vi "JSON Key Search.vi"(9 "offset (0)":i32, 10 "Key":string, 11 "JSON":string) -> (1 "offset of match":i32, 2 "JSON Type":T1, 3 "Value":string)   [LabVIEW 2013, in "LV JSON.lvlib"]
doc: "Search JSON string for Key name and return corresponding value and the JSON type of the value."
uses:
  LV JSON.lvlib
  controls/JSON type.ctl
  <vilib>/Utility/error.llb/Trim Whitespace.vi
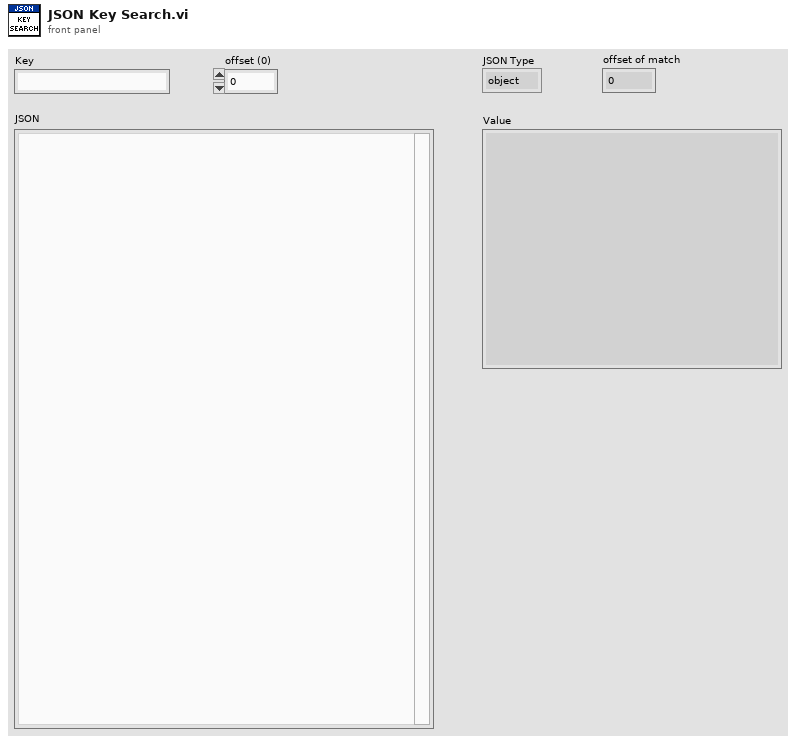
[diagram p1: front panel]
types:
  T1 = typedef "LV JSON.lvlib/JSON type.ctl" = enum16{"object", "array", "number", "string", "boolean", "null"}
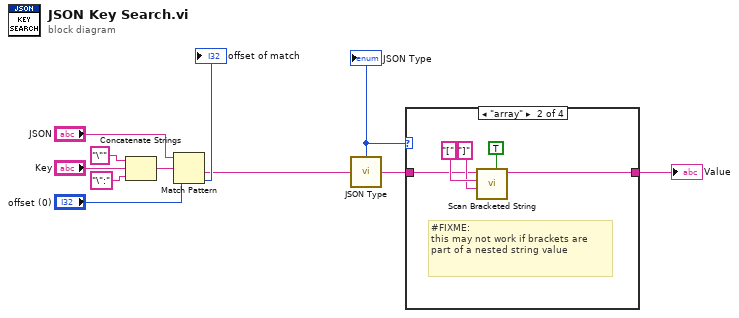
[diagram p0: block diagram]
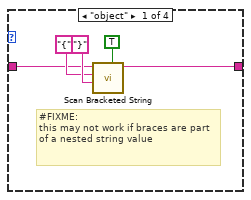
[diagram p2: hidden frame]
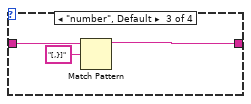
[diagram p3: hidden frame]
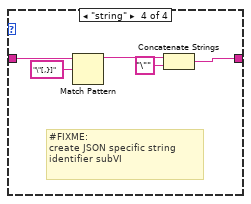
[diagram p4: hidden frame]
diagram:
  n1 = Concatenate Strings("\"" ("string"), "Key", "\":" ("string")) -> (w8:string)
  n2 = Match Pattern(string="JSON", regular expression=w8, offset (0)="offset (0)") -> (after substring=w1:string, offset past match=→"offset of match":i32)  [unwired: 2 out]
  n3 = call "JSON Type.vi"("JSON Value"=w1) -> ("JSON Value Type"=w7:T1, "JSON Value Out (dup)"=w5:string)
  "JSON Type" <- w7
  n4 = case shown="\"array\"" w7 {
    tunnel: w5 -> [w13 w18 w24 w28]
    tunnel: [w12 w17 w22 w26] -> w4
    frame "object" {
      # "#FIXME:\nthis may not work if braces are part of a nested string value"
      n5 = call "Scan Bracketed String.vi"("Include Brackets (F)"=TRUE, "End"="}", "Start"="{", "String"=w13) -> ("Substring"=w12:string)  [unwired: 5 in, 2 out]
    }
    frame "array" {
      # "#FIXME:\nthis may not work if brackets are part of a nested string value"
      n6 = call "Scan Bracketed String.vi"("Include Brackets (F)"=TRUE, "End"="]", "Start"="[", "String"=w18) -> ("Substring"=w17:string)  [unwired: 5 in, 2 out]
    }
    frame "number", Default {
      n7 = Match Pattern(string=w24, regular expression="[,}]" ("search string/char (-)")) -> (before substring=w22:string)  [unwired: 1 in, 3 out]
    }
    frame "string" {
      # "#FIXME:\ncreate JSON specific string identifier subVI"
      n8 = Match Pattern(string=w28, regular expression="\"[,}]" ("search string/char (-)")) -> (before substring=w27:string)  [unwired: 1 in, 3 out]
      n9 = Concatenate Strings(w27, "\"" ("string")) -> (w26:string)
    }
  }
  "Value" <- w4
